vi "DOTNET - Bitmap Pointer to LV_Image.vi"(0 "Bitmap":refnum<k24>, 11 "error in (no error)":errorcluster) -> (4 "Bitmap dup":refnum<k24>, 8 "LV_Image":T1, 10 "Image (U32)":u32[][](array[numeric]), 15 "error out":errorcluster)   [LabVIEW 2014]
uses:
  System.Drawing
  <vilib>/picture/picture.llb/imagedata.ctl
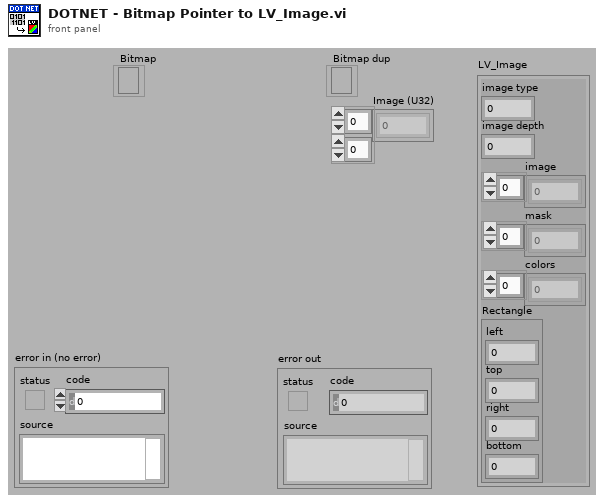
[diagram p1: front panel]
types:
  T1 = typedef "imagedata.ctl" = cluster{"image type":i32, "image depth":i32, "image":u8[], "mask":u8[], "colors":u32[], "Rectangle":cluster{"left":i16, "top":i16, "right":i16, "bottom":i16}}
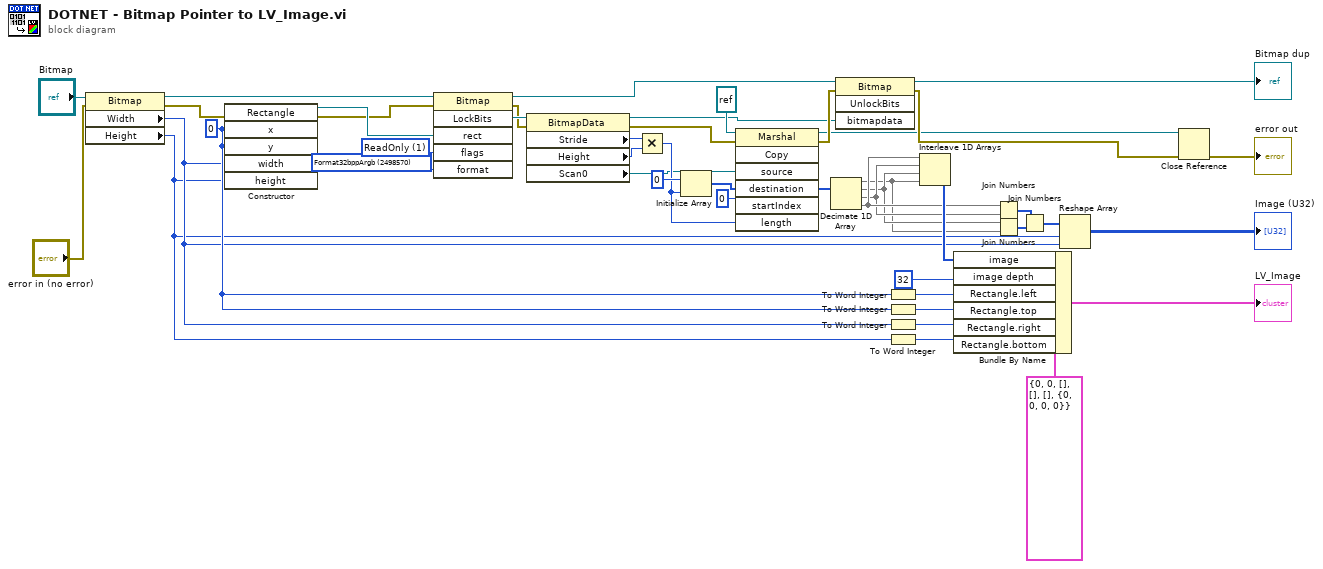
[diagram p0: block diagram]
diagram:
  w20 = 0 ("x")
  w41 = 2498570 items=["DontCare, Undefined"=0, "Max"=15, "Indexed"=65536, "Gdi"=131072, "Format16bppRgb555"=135173, "Format16bppRgb565"=135174, "Format24bppRgb"=137224, "Format32bppRgb"=139273, "Format1bppIndexed"=196865, "Format4bppIndexed"=197634, "Format8bppIndexed"=198659, "Alpha"=262144, "Format16bppArgb1555"=397319, "PAlpha"=524288, "Format32bppPArgb"=925707, "Extended"=1048576, "Format16bppGrayScale"=1052676, "Format48bppRgb"=1060876, "Format64bppPArgb"=1851406, "Canonical"=2097152, "Format32bppArgb"=2498570, "Format64bppArgb"=3424269] ("format")
  w42 = 1 items=["ReadOnly"=1, "WriteOnly"=2, "ReadWrite"=3, "UserInputBuffer"=4] ("flags")
  n1 = property class="Bitmap"(reference="Bitmap", error in="error in (no error)") -> (reference out=w43:refnum<k24>, error out=w46:errorcluster, "Width"=w10:i32, "Height"=w9:i32)
  n2 = constructor class="Rectangle"(error in=w46, "x"=w20, "y"=w20, "width"=w10, "height"=w9) -> (reference out=w45:refnum<k24>, error out=w44:errorcluster)  [unwired: 2 in, 5 out]
  n3 = invoke class="Bitmap" method="LockBits"(reference=w43, error in=w44, "rect"=w45, "flags"=w42, "format"=w41) -> (reference out=w35:refnum<k24>, error out=w39:errorcluster, "LockBits"=w40:refnum<k24>)  [unwired: 1 in, 3 out]
  n4 = property class="BitmapData"(reference=w40, error in=w39) -> (reference out=w4:refnum<k24>, error out=w33:errorcluster, "Stride"=w38:i32, "Height"=w37:i32, "Scan0"=w3:refnum<k24>)
  n5 = Multiply(x=w38, y=w37) -> (x*y=w30:i32)
  n6 = Initialize Array(u8 0 ("element"), w30) -> (w32:u8[])
  n7 = invoke class="Marshal" method="Copy"(reference=refnum<k24> refnum ("reference out"), error in=w33, "source"=w3, "destination"=w32, "startIndex"=0, "length"=w30) -> (reference out=w1:refnum<k24>, error out=w29:errorcluster, "destination"=w24:u8[])  [unwired: 1 in, 4 out]
  n8 = Decimate 1D Array(w24) -> (w5:u8[], w6:u8[], w7:u8[], w8:u8[])
  n9 = invoke class="Bitmap" method="UnlockBits"(reference=w35, error in=w29, "bitmapdata"=w4) -> (reference out=→"Bitmap dup":refnum<k24>, error out=w2:errorcluster)  [unwired: 1 in, 2 out]
  n10 = To Word Integer(number=w20) -> (16bit integer=w19:i16)
  n11 = To Word Integer(number=w20) -> (16bit integer=w18:i16)
  n12 = To Word Integer(number=w10) -> (16bit integer=w17:i16)
  n13 = To Word Integer(number=w9) -> (16bit integer=w16:i16)
  n14 = Interleave 1D Arrays(w8, w7, w6, w5) -> (w12:u8[])
  n15 = Bundle By Name(cluster=T1 {"image type"=0, "image depth"=0, "image"=[], "mask"=[], "colors"=[], "Rectangle"={"left"=0, "top"=0, "right"=0, "bottom"=0}} ("LV_Image"), "image"=w12, "image depth"=32, "Rectangle.left"=w19, "Rectangle.top"=w18, "Rectangle.right"=w17, "Rectangle.bottom"=w16) -> (→"LV_Image":T1)
  n16 = Join Numbers(hi=w8, lo=w7) -> ((hi.lo)=w14:u16[])
  n17 = Join Numbers(hi=w6, lo=w5) -> ((hi.lo)=w15:u16[])
  n18 = Join Numbers(hi=w14, lo=w15) -> ((hi.lo)=w13:u32[])
  n19 = Reshape Array(w13, w9, w10) -> (→"Image (U32)":u32[][])
  n20 = Close Reference(reference=w1, error in (no error)=w2) -> (error out=→"error out":errorcluster)
